vi "Close.vi"(8 "error in (no error)":errorcluster, 11 "CryoCoolerAVC in":refnum<class "CryoCoolerAVC.lvclass">) -> (0 "error out":errorcluster, 3 "CryoCoolerAVC out":refnum<class "CryoCoolerAVC.lvclass">)   [LabVIEW 2024, in "CryoCoolerAVC.lvclass"]
uses:
  CryoCoolerAVC.lvclass
  CryoCoolerAVC.lvclass/CryoCoolerAVC.ctl
  Cryo Cooler.lvclass
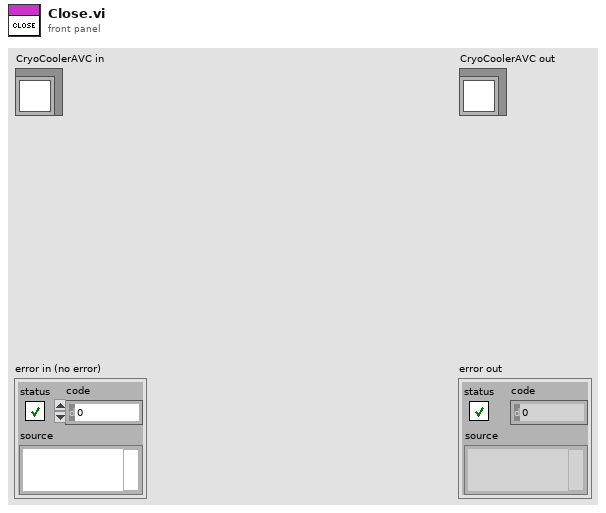
[diagram p1: front panel]
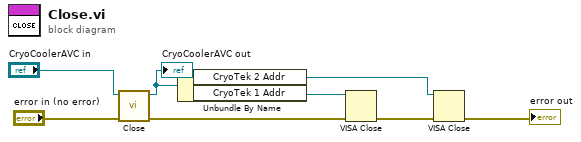
[diagram p0: block diagram]
diagram:
  n1 = call-parent "Close.vi"("error in (no error)"="error in (no error)", "Cryo Cooler in"="CryoCoolerAVC in") -> ("error out"=w4:errorcluster, "Cryo Cooler out"=w6:refnum<class "CryoCoolerAVC.lvclass">)  [unwired: 8 in]
  "CryoCoolerAVC out" <- w6
  n2 = Unbundle By Name(w6) -> ("CryoTek 2 Addr"=w2:refnum<visa-resource-name>, "CryoTek 1 Addr"=w5:refnum<visa-resource-name>)
  n3 = VISA Close(VISA resource name=w5, error in (no error)=w4) -> (error out=w3:errorcluster)
  n4 = VISA Close(VISA resource name=w2, error in (no error)=w3) -> (error out=→"error out":errorcluster)
